vi "Unit Test - copy state.vi"() -> (3 "Array":T1(array[cluster])=[{"state"="Idle", "error out"={"status"=FALSE, "code"=0, "source"=""}, "Execution:State"=enum."Idle"}, {"state"="CSM Documentation", "error out"={"status"=FALSE, "code"=0, "source"=""}, "Execution:State"=enum."Idle"}, {"state"="VI Reference", "error out"={"status"=FALSE, "code"=0, "source"=""}, "Execution:State"=enum."Idle"}, {"state"="Error Handler", "error out"={"status"=FALSE, "code"=0, "source"=""}, "Execution:State"=enum."Bad"}, {"state"="Critical Error", "error out"={"status"=FALSE, "code"=0, "source"=""}, "Execution:State"=enum."Idle"}, {"state"="Target Timeout Error", "error out"={"status"=FALSE, "code"=0, "source"=""}, "Execution:State"=enum."Idle"}, {"state"="Target Error", "error out"={"status"=FALSE, "code"=0, "source"=""}, "Execution:State"=enum."Idle"}, {"state"="Async Response", "error out"={"status"=FALSE, "code"=0, "source"=""}, "Execution:State"=enum."Idle"}, {"state"="Response", "error out"={"status"=FALSE, "code"=0, "source"=""}, "Execution:State"=enum."Idle"}, {"state"="Async Message Posted", "error out"={"status"=FALSE, "code"=0, "source"=""}, "Execution:State"=enum."Idle"}, {"state"="Initialize Core Data", "error out"={"status"=FALSE, "code"=0, "source"=""}, "Execution:State"=enum."Idle"}, {"state"="Exit", "error out"={"status"=FALSE, "code"=0, "source"=""}, "Execution:State"=enum."Idle"}, {"state"="Data: Initialize", "error out"={"status"=FALSE, "code"=0, "source"=""}, "Execution:State"=enum."Idle"}, {"state"="Data: Update Indicators", "error out"={"status"=FALSE, "code"=0, "source"=""}, "Execution:State"=enum."Idle"}, {"state"="Data: Cleanup", "error out"={"status"=FALSE, "code"=0, "source"=""}, "Execution:State"=enum."Idle"}, {"state"="Macro: Initialize", "error out"={"status"=FALSE, "code"=0, "source"=""}, "Execution:State"=enum."Idle"}, {"state"="Macro: Exit", "error out"={"status"=FALSE, "code"=0, "source"=""}, "Execution:State"=enum."Idle"}, {"state"="API: API1", "error out"={"status"=FALSE, "code"=0, "source"=""}, "Execution:State"=enum."Idle"}, {"state"="API: API2", "error out"={"status"=FALSE, "code"=0, "source"=""}, "Execution:State"=enum."Idle"}, {"state"="Action: action1", "error out"={"status"=FALSE, "code"=0, "source"=""}, "Execution:State"=enum."Idle"}, {"state"="Action: action2", "error out"={"status"=FALSE, "code"=0, "source"=""}, "Execution:State"=enum."Idle"}])   [LabVIEW 2017, in "testcase-csmhelper.lvclass"]
uses:
  testcase-csmhelper.lvclass
  src/user.lib/_NEVSTOP/Communicable State Machine(CSM)/_csmHelper/CSM-Helper.lvclass/CSM-Helper.ctl
  src/user.lib/_NEVSTOP/Communicable State Machine(CSM)/_csmHelper/Properties/Read VI Ref.vi
  src/user.lib/_NEVSTOP/Communicable State Machine(CSM)/_csmHelper/API/Create From VI Reference.vi
  src/user.lib/_NEVSTOP/Communicable State Machine(CSM)/_csmHelper/Properties/Read States.vi
  src/user.lib/_NEVSTOP/Communicable State Machine(CSM)/_csmHelper/API/Start Undo.vi
  src/user.lib/_NEVSTOP/Communicable State Machine(CSM)/_csmHelper/API/Copy State.vi
  src/user.lib/_NEVSTOP/Communicable State Machine(CSM)/_csmHelper/API/Stop Undo.vi
  src/user.lib/_NEVSTOP/Communicable State Machine(CSM)/_csmHelper/API/Undo.vi
  src/user.lib/_NEVSTOP/Communicable State Machine(CSM)/_csmHelper/API/Destroy.vi
  src/user.lib/_NEVSTOP/Communicable State Machine(CSM)/_csmHelper/CSM-Helper.lvclass
  src/user.lib/_NEVSTOP/Communicable State Machine(CSM)/_csmHelper/API/Open Block Diagram.vi
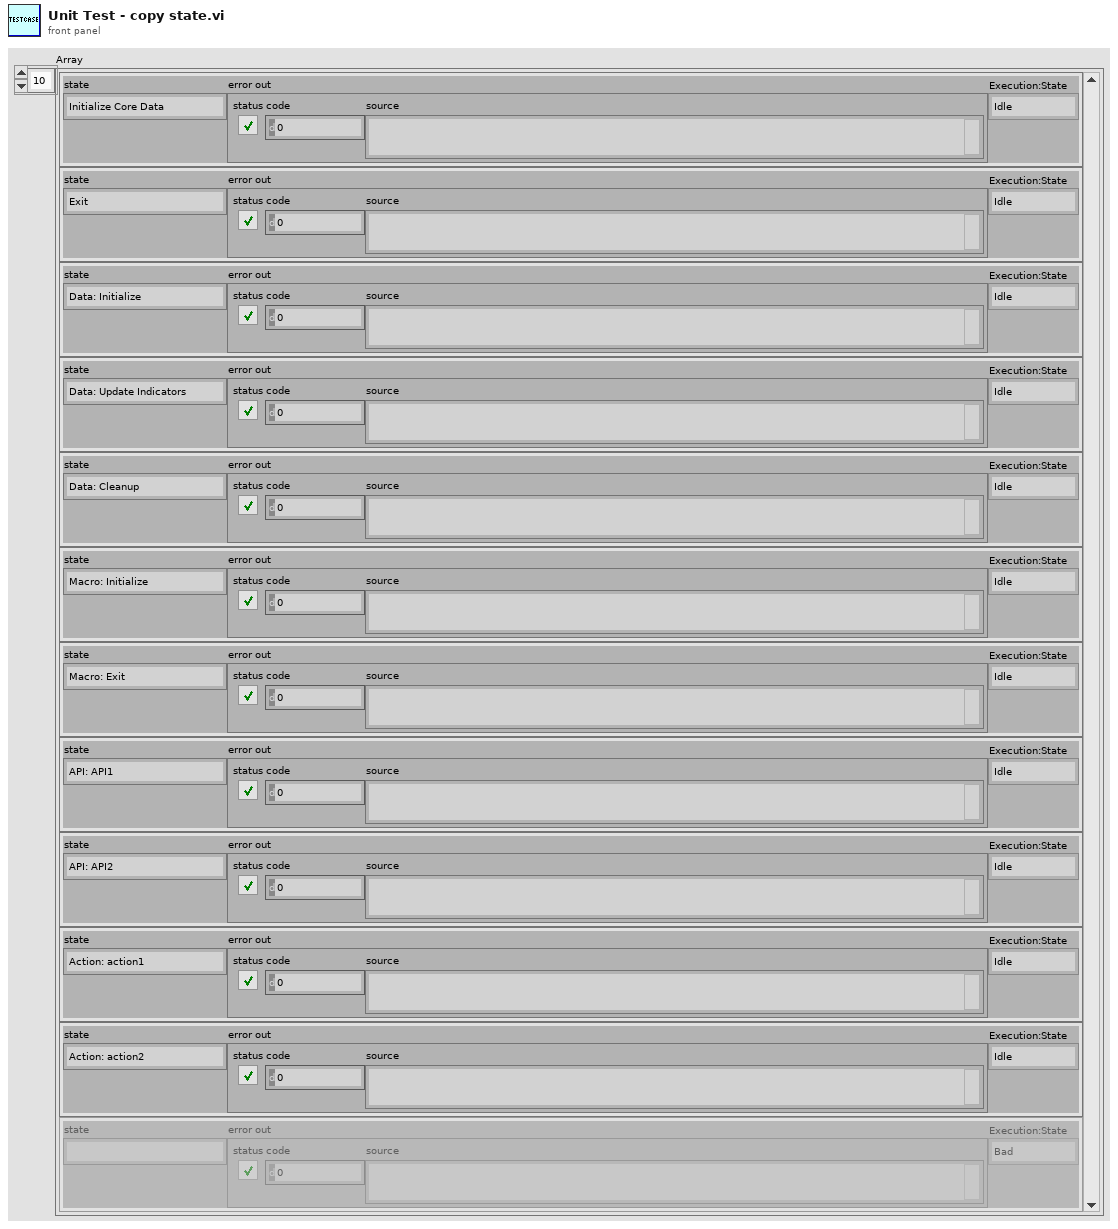
[diagram p1: front panel]
types:
  T1 = cluster{"state":string, "error out":errorcluster, "Execution:State":enum32{"Bad", "Idle", "Run top level", "Running"}}[]
  T2 = enum32{"Bad", "Idle", "Run top level", "Running"}
  T3 = cluster{string, "error out":errorcluster, "Exec.State":enum32{"Bad", "Idle", "Run top level", "Running"}}
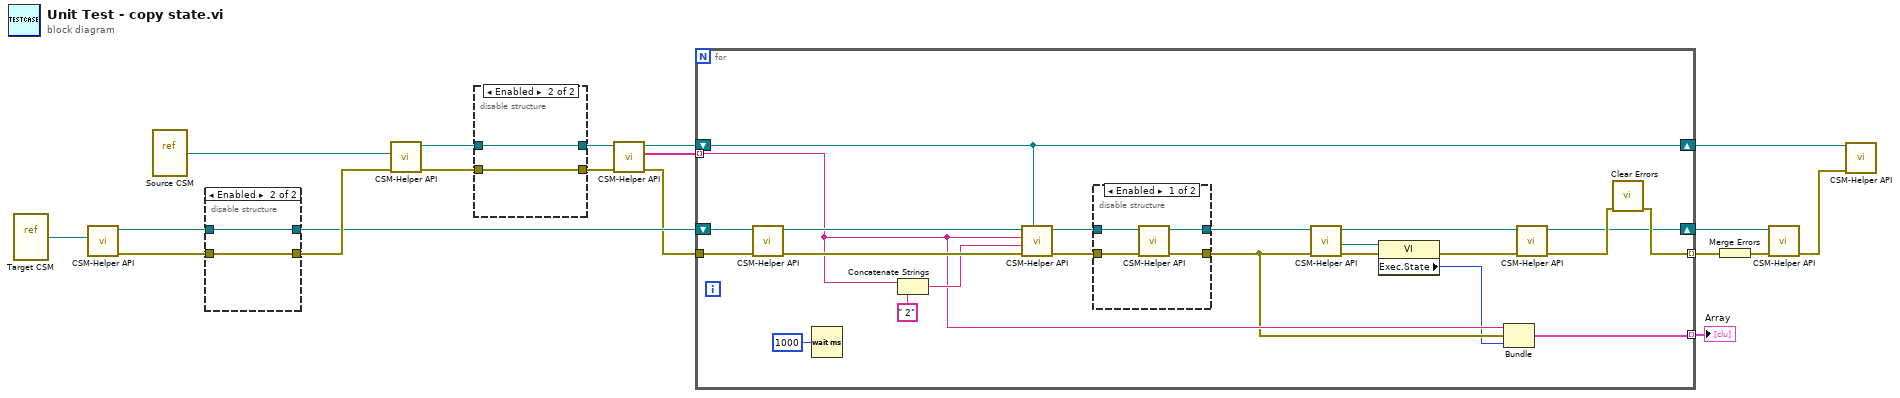
[diagram p0: block diagram]
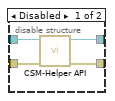
[diagram p2: hidden frame]
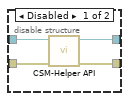
[diagram p3: hidden frame]
diagram:
  n1 = vi-ref "Target CSM.vi"() -> (w18:refnum<vi>)
  n2 = call-poly "CSM-Helper API.vi"("VI"=w18) -> ("error out"=w15:errorcluster, "CSM-Helper.lvclass"=w14:refnum<class "CSM-Helper.lvclass">)  [unwired: 9 in]
  n3 = vi-ref "Source CSM.vi"() -> (w19:refnum<vi>)
  n4 = disable-structure shown="Enabled" {
    disable-tunnel: w15 -> [w23 w25]
    disable-tunnel: w14 -> [w22 w24]
    disable-tunnel: [w21 w25] -> w9
    disable-tunnel: [w20 w24] -> w8
    frame Disabled {
      n5 = call-poly "CSM-Helper API.vi"("error in (no error)"=w23, "CSM-Helper in"=w22) -> ("error out"=w21:errorcluster, "CSM-Helper out"=w20:refnum<class "CSM-Helper.lvclass">)  [unwired: 8 in]
    }
    frame Enabled {
    }
  }
  n6 = call-poly "CSM-Helper API.vi"("error in (no error)"=w9, "VI"=w19) -> ("error out"=w12:errorcluster, "CSM-Helper.lvclass"=w13:refnum<class "CSM-Helper.lvclass">)  [unwired: 8 in]
  n7 = disable-structure shown="Enabled" {
    disable-tunnel: w13 -> [w29 w31]
    disable-tunnel: w12 -> [w28 w30]
    disable-tunnel: [w27 w30] -> w11
    disable-tunnel: [w26 w31] -> w10
    frame Disabled {
      n8 = call-poly "CSM-Helper API.vi"("error in (no error)"=w28, "CSM-Helper in"=w29) -> ("error out"=w27:errorcluster, "CSM-Helper out"=w26:refnum<class "CSM-Helper.lvclass">)  [unwired: 8 in]
    }
    frame Enabled {
    }
  }
  n9 = call-poly "CSM-Helper API.vi"("error in (no error)"=w11, "CSM-Helper in"=w10) -> ("error out"=w7:errorcluster, "Value"=w3:string[], "CSM-Helper out"=w6:refnum<class "CSM-Helper.lvclass">)  [unwired: 7 in]
  n10 = for {
    shift-right: [w39] -> w17
    shift-left: w8 -> [w52]
    shift-right: [w47] -> w4
    shift-left: w6 -> [w47]
    tunnel: w3 -> [w43] mode=indexing
    tunnel: w7 -> [w51]
    tunnel: [w44] -> w16 mode=indexing
    tunnel: [w42] -> w1 mode=indexing
    n11 = call-poly "CSM-Helper API.vi"("error in (no error)"=w51, "CSM-Helper in"=w52) -> ("error out"=w50:errorcluster, "CSM-Helper out"=w49:refnum<class "CSM-Helper.lvclass">)  [unwired: 8 in]
    n12 = Wait (ms)(milliseconds to wait=u32 1000) -> ()  [unwired: 1 out]
    n13 = Concatenate Strings(w43, " 2" ("string")) -> (w46:string)
    n14 = call-poly "CSM-Helper API.vi"("SourceCSM"=w47, "error in (no error)"=w50, "New(Empty to Use same Name)"=w46, "Case"=w43, "CSM-Helper.lvclass"=w49) -> ("error out"=w48:errorcluster, "CSM-Helper out 2"=w53:refnum<class "CSM-Helper.lvclass">)  [unwired: 5 in]
    n15 = disable-structure shown="Enabled" {
      disable-tunnel: [w57 w59] -> w37
      disable-tunnel: w48 -> [w56 w58]
      disable-tunnel: [w55 w58] -> w38
      disable-tunnel: w53 -> [w54 w59]
      frame Enabled {
        n16 = call-poly "CSM-Helper API.vi"("error in (no error)"=w56, "CSM-Helper in"=w54) -> ("error out"=w55:errorcluster, "CSM-Helper out"=w57:refnum<class "CSM-Helper.lvclass">)  [unwired: 8 in]
      }
      frame Disabled {
      }
    }
    n17 = call-poly "CSM-Helper API.vi"("error in (no error)"=w38, "CSM-Helper in"=w37) -> ("error out"=w35:errorcluster, "VI"=w33:refnum<vi>, "CSM-Helper out"=w36:refnum<class "CSM-Helper.lvclass">)  [unwired: 7 in]
    n18 = property class="VI"(reference=w33, error in=w35) -> (error out=w34:errorcluster, "Exec.State"=w32:T2)  [unwired: 1 out]
    n19 = Bundle(w43, "error out"=w38, "Exec.State"=w32) -> (w42:T3)  [unwired: 1 in]
    n20 = call-poly "CSM-Helper API.vi"("error in (no error)"=w34, "CSM-Helper in"=w36) -> ("error out"=w40:errorcluster, "CSM-Helper out"=w39:refnum<class "CSM-Helper.lvclass">)  [unwired: 8 in]
    n21 = call <vilib>:"Clear Errors.vi"("error in (no error)"=w40) -> ("error out"=w44:errorcluster)  [unwired: 5 in, 1 out]
  }
  "Array" <- w1
  n22 = Merge Errors(w16) -> (w2:errorcluster)
  n23 = call-poly "CSM-Helper API.vi"("error in (no error)"=w2, "CSM-Helper in"=w17) -> ("error out"=w5:errorcluster)  [unwired: 8 in, 1 out]
  n24 = call-poly "CSM-Helper API.vi"("error in (no error)"=w5, "CSM-Helper in"=w4) -> ()  [unwired: 8 in, 2 out]
